vi "UV-VIs SetADChannelSD.vi"(3 "error in (no error)":errorcluster, 4 "channel":i32, 5 "Control in":refnum<class "CCD_camera.lvclass">) -> (0 "error out":errorcluster, 1 "DLL error code":u32, 2 "Control out":refnum<class "CCD_camera.lvclass">)   [LabVIEW 2015, in "CCD_camera.lvclass"]
doc: "This function will set the AD channel to one of the possible A-Ds of the system. It will be used for subsequent acquisitions.\n\n<B>Parameter:</B>\nindex - the channel to be used\n Valid values: 0 to <B>GetNumberADChannels</B>-1\n\n<B>Error codes:</B>\nDRV_SUCCESS - AD channel set.\nDRV_P1INVALID - Index is out off range."
uses:
  CCD_camera.lvclass
  Detector.lvclass/Detector.ctl
  Detector.lvclass
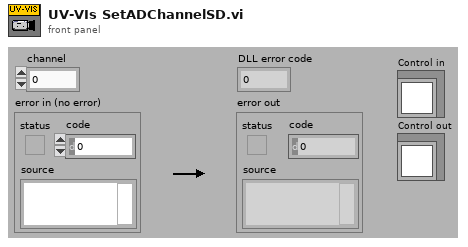
[diagram p1: front panel]
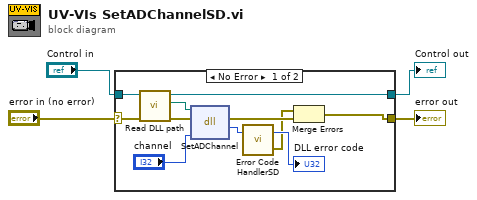
[diagram p0: block diagram]
diagram:
  n1 = case shown="No Error" "error in (no error)" {
    selector: "error in (no error)" -> [w12 w17]
    tunnel: [w7 w17] -> w3
    tunnel: [w5 w16] -> w2
    tunnel: "Control in" -> [w6 w16]
    frame No Error {
      n2 = call "Read DLL path.vi"("error in (no error)"=w12, "Detector in"=w6) -> ("error out"=w11:errorcluster, "DLL path"=w10:path, "Detector out"=w5:refnum<class "CCD_camera.lvclass">)  [unwired: 7 in]
      n3 = dll-call lib="S:/TRANCON/DLL/Atmcd32d.dll" fn="SetADChannel"(path in=w10, error in=w11, "channel"="channel") -> (error out=w9:errorcluster, "return type"=w15:u32)  [unwired: 2 in, 1 out]
      n4 = call "Error Code HandlerSD.vi"("DLL error code"=w15) -> ("error out"=w8:errorcluster, "dup DLL error code"=→"DLL error code":u32)  [unwired: 1 in]
      n5 = Merge Errors(w8, w9) -> (w7:errorcluster)
    }
    frame Error {
    }
  }
  "error out" <- w3
  "Control out" <- w2
